vi "Write Roles.vi"(8 "error in (no error)":errorcluster, 10 "Roles":T1, 11 "SimpleBallPlacementAllyPlay in":refnum<class "SimpleBallPlacementAllyPlay.lvclass">) -> (0 "error out":errorcluster, 3 "SimpleBallPlacementAllyPlay out":refnum<class "SimpleBallPlacementAllyPlay.lvclass">)   [LabVIEW 2020, in "SimpleBallPlacementAllyPlay.lvclass"]
uses:
  SimpleBallPlacementAllyPlay.lvclass
  RolesSimpleBallPlacementAllyPlay.ctl
  BallPlacementEnemyRole_class/BallPlacementEnemyRole.lvclass
  SimpleBallPlacementAllyPlay.lvclass/SimpleBallPlacementAllyPlay.ctl
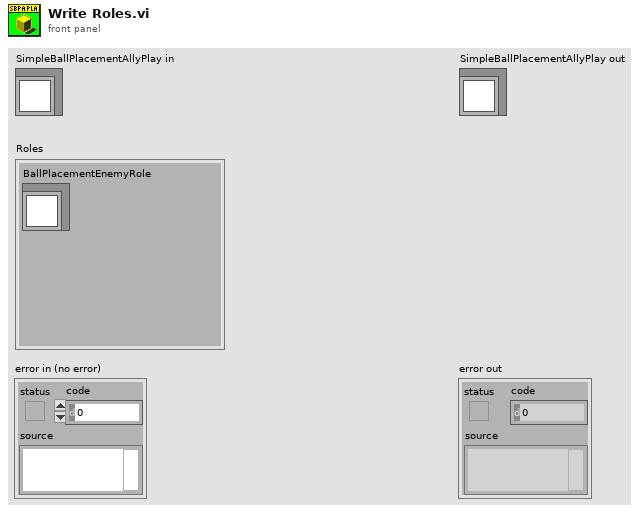
[diagram p1: front panel]
types:
  T1 = typedef "SimpleBallPlacementAllyPlay.lvclass/RolesSimpleBallPlacementAllyPlay.ctl" = cluster{"BallPlacementEnemyRole":refnum<class "BallPlacementEnemyRole.lvclass">}
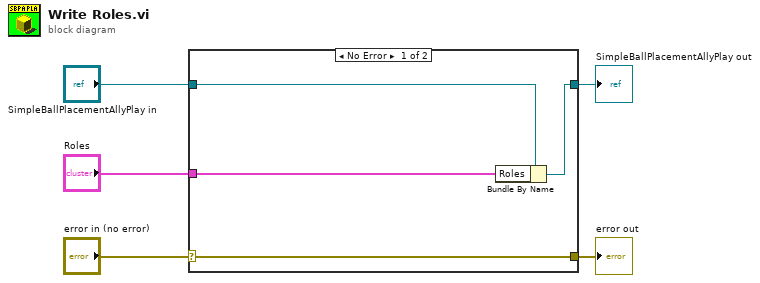
[diagram p0: block diagram]
diagram:
  n1 = case shown="No Error" "error in (no error)" {
    selector: "error in (no error)" -> [w9 w10]
    tunnel: [w9 w10] -> w4
    tunnel: [w7 w11] -> w2
    tunnel: "SimpleBallPlacementAllyPlay in" -> [w8 w11]
    tunnel: "Roles" -> [w6 _]
    frame No Error {
      n2 = Bundle By Name(cluster=w8, "Roles"=w6) -> (w7:refnum<class "SimpleBallPlacementAllyPlay.lvclass">)
    }
    frame Error {
    }
  }
  "error out" <- w4
  "SimpleBallPlacementAllyPlay out" <- w2
